vi "Stream Waveforms.vi"(9 "Stop":bool, 10 "Waveform Paths":string[](array[string])=["Targets/Controller/Hardware/Chassis/DAQ/PXI1Slot2/Analog Input/AI0", "Targets/Controller/Hardware/Chassis/DAQ/PXI1Slot2/Analog Input/AI1", "Targets/Controller/Hardware/Chassis/DAQ/PXI1Slot2/Analog Input/AI2", "Targets/Controller/Hardware/Chassis/DAQ/PXI1Slot2/Analog Input/AI3"]) -> (0 "error out":errorcluster={"status"=TRUE, "code"=-2501, "source"="TDMS Close in Stream Waveforms.vi"})   [LabVIEW 2015]
uses:
  NationalInstruments.VeriStand.ClientAPI
  <vilib>/NI Veristand/Execution/Workspace/NI VeriStand - Set Single Channel Value.vi
  <vilib>/NI Veristand/Execution/WaveformStreaming/NI_VS Waveform Streaming Interface.lvlib
  <vilib>/Analysis/NI_AALBase.lvlib
  <vilib>/NI Veristand/Execution/Workspace/NI_VS Workspace ExecutionAPI.lvlib
panel:
  in  "Waveform Task Trigger Channel":string="Targets/Controller/Hardware/Chassis/DAQ/Waveform Tasks/DAQ1/Triggers/Start Trigger"
  out "data":waveform(dbl)[](graph)
  in  "Samples to View":i64(slide)=1010 scale=300000.0..4000000.0
  in  "Offset":i64=100
  in  "Log File Path":path=path "c:/logs/log.tdms"
  out "AI2 Samples":u64
  out "AI2 offset from start (samples)":u64
  out "AI1 Samples":u64
  out "AI1 offset from start (samples)":u64
  out "AI0 Samples":u64
  out "AI0 offset from start (samples)":u64
  out "AI3 Samples":u64
  out "AI3 offset from start (samples)":u64
  out "Loop Rate Histogram":T1(graph)={"X Values"=[0.20333589539806454, 0.6100044137911523, 1.0166729321842403, 1.423341450577328, 1.830009968970416, 2.2366784873635037, 2.6433470057565915, 3.0500155241496794, 3.456684042542767, 3.863352560935855, 4.270021079328943, 4.6766895977220315, 5.08335811611512, 5.490026634508208, 5.896695152901296, 6.303363671294385, 6.710032189687473, 7.116700708080561, 7.523369226473649, 7.930037744866738, 8.336706263259826, 8.743374781652914, 9.150043300046002, 9.55671181843909, 9.963380336832179, 10.370048855225267, 10.776717373618355, 11.183385892011444, 11.590054410404532, 11.99672292879762, 12.403391447190709, 12.810059965583797, 13.216728483976885, 13.623397002369973, 14.030065520763062, 14.43673403915615, 14.843402557549238, 15.250071075942326, 15.656739594335415, 16.063408112728503, 16.47007663112159, 16.876745149514676, 17.283413667907762, 17.69008218630085, 18.096750704693935, 18.503419223087022, 18.91008774148011, 19.316756259873195, 19.72342477826628, 20.130093296659368], "Histogram: h(x)"=[1, 0, 0, 0, 0, 0, 0, 0, 0, 0, 0, 0, 0, 0, 0, 0, 0, 0, 0, 0, 0, 0, 0, 1, 0, 0, 1, 0, 0, 0, 1, 2, 3, 2, 1, 4, 4, 2, 1, 2, 0, 4, 2, 7, 7, 10, 8, 37, 248, 438]}
  out "Elapsed time":dbl
  out "Loop Rate (Hz)":dbl=19.610227107632454
  # "1. Run this VI after the VeriStand Engine is running on the target."
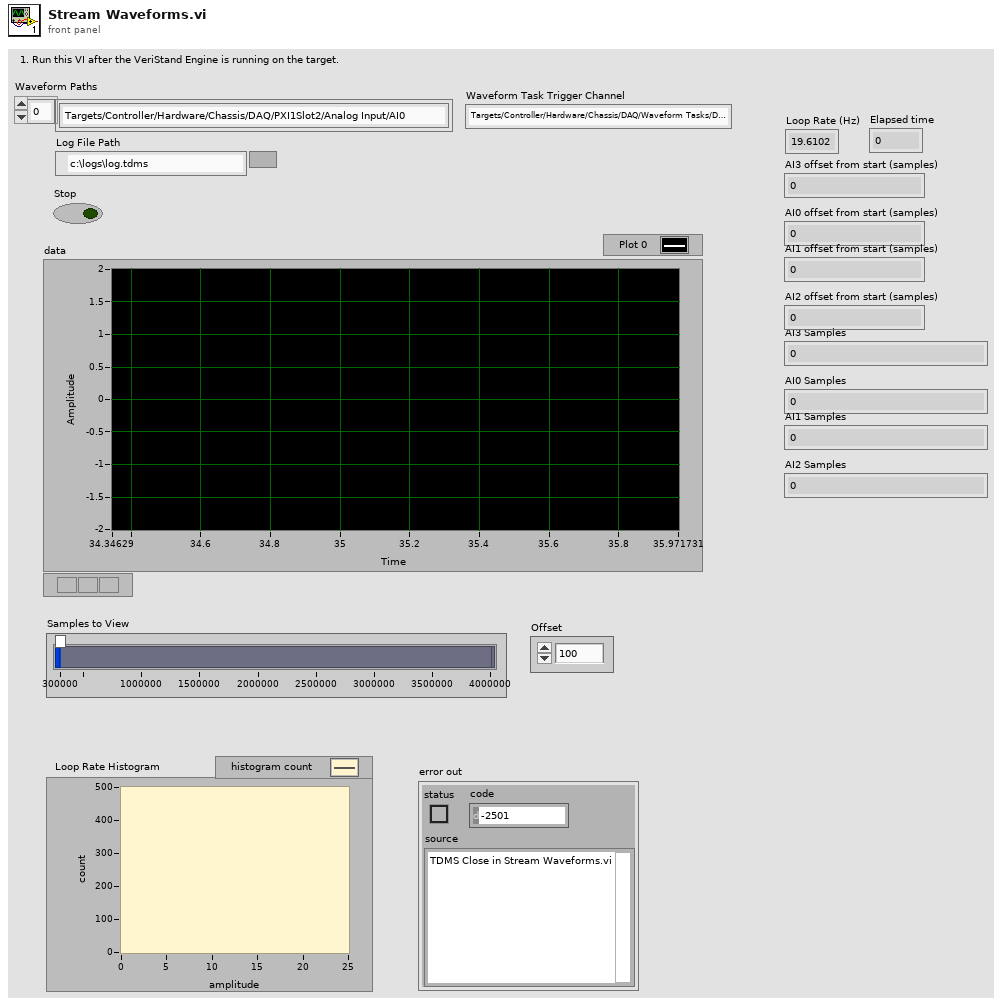
[diagram p1: front panel]
types:
  T1 = cluster{"X Values":dbl[], "Histogram: h(x)":i32[]}
  T2 = enum16{"open", "open or create", "create or replace", "create", "open (read-only)"}
  T3 = typedef "NI_VS Workspace ExecutionAPI.lvlib/WorkspaceAPI.ctl" = refnum<k24>
  T4 = typedef "NI_VS Waveform Streaming Interface.lvlib/WaveformStreamSpecification.ctl" = refnum<k24>
  T5 = typedef "NI_VS Waveform Streaming Interface.lvlib/WaveformStreamingAPI.ctl" = refnum<k24>
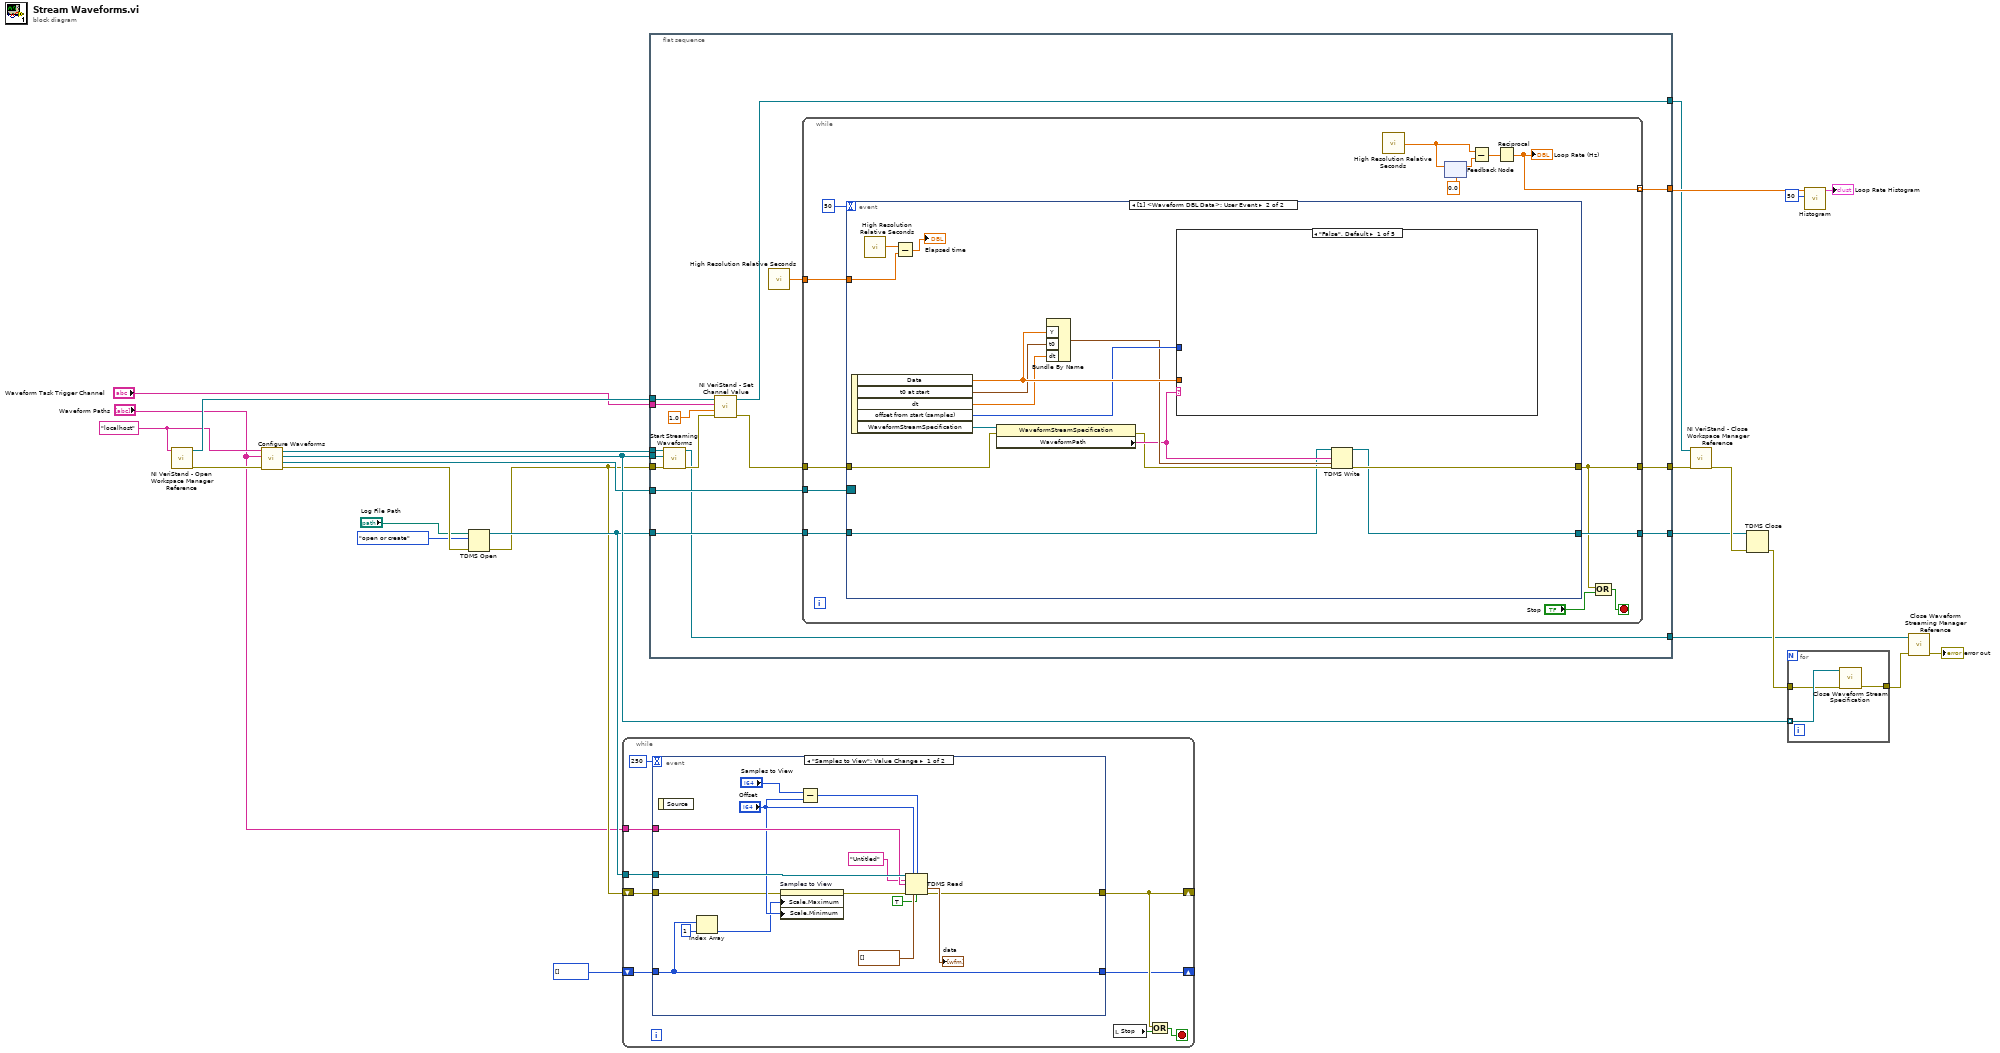
[diagram p0: block diagram]
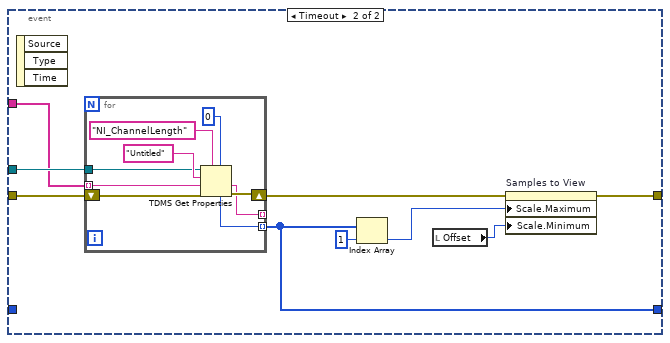
[diagram p2: hidden frame]
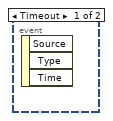
[diagram p3: hidden frame]
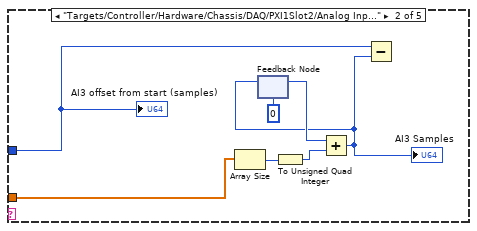
[diagram p4: hidden frame]
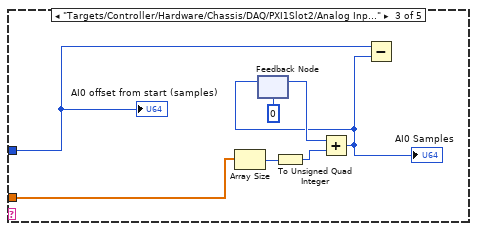
[diagram p5: hidden frame]
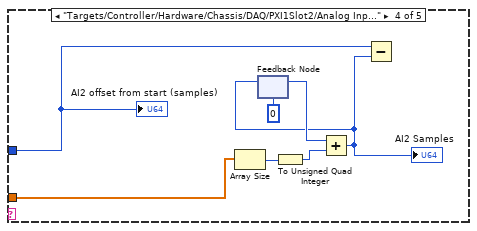
[diagram p6: hidden frame]
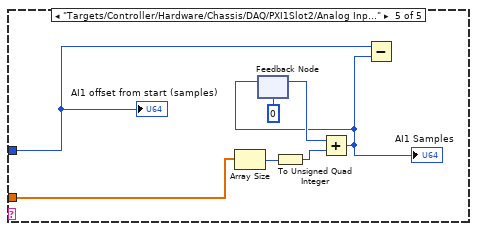
[diagram p7: hidden frame]
diagram:
  w16 = "localhost" ("Gateway IP Address (\"\": localhost)")
  n1 = call <vilib>:"NI VeriStand - Open Workspace Manager Reference.vi"("Gateway IP Address (\"\": localhost)"=w16) -> ("error out"=w17:errorcluster, "WorkspaceManager"=w20:T3)  [unwired: 9 in]
  n2 = call "Configure Waveforms.vi"("error in (no error)"=w17, "Waveform paths"="Waveform Paths", "Gateway IP Address (\"\": localhost)"=w16) -> ("error out"=w12:errorcluster, "waveform data event registration (DBL)"=w14:refnum<event-registration>, "WaveformStreamSpecifications"=w13:T4[], "WaveformStreaming out"=w15:T5)  [unwired: 5 in]
  n3 = TDMS Open(8:w12, 10:T2."open or create" ("operation (0:open)"), 11:"Log File Path") -> (0:w3:errorcluster, 3:w4:refnum<k34>)  [unwired: 4 in]
  n4 = while {
    tunnel: w4 -> [w34]
    tunnel: "Waveform Paths" -> [w33]
    shift-right: [w28] -> _
    shift-left: w3 -> [w32]
    shift-right: [w26] -> _
    shift-left: u64[] [] -> [w31]
    stop <- w30 stop-if-true
    n5 = event shown="[0] \"Samples to View\": Value Change" {
      selector: _ -> [_ _]
      dyn-events: _ -> [_ _]
      timeout: 250 -> [_ _]
      tunnel: w34 -> [w49 w57]
      tunnel: w33 -> [w48 w56]
      tunnel: w32 -> [w44 w58]
      tunnel: w31 -> [w35 _]
      tunnel: [w37 w52] -> w28
      tunnel: [w35 w54] -> w26
      event "Samples to View": Value Change {
        n6 = event-data() -> ()  [unwired: 1 in, 1 out]
        n7 = Index Array(array=w35, index=1) -> (element=w42:u64)
        n8 = property on="Samples to View" class="Slide (strict)"(error in=w44, "Scale.Maximum"=w42, "Scale.Minimum"="Offset") -> (error out=w43:errorcluster)  [unwired: 1 in, 1 out]
        n9 = Subtract(x="Samples to View", y="Offset") -> (x-y=w46:i64)
        n10 = TDMS Read(0:w49, 1:"Offset", 2:w46, 5:"Untitled" ("group name in"), 7:w48, 11:w43, 12:waveform(dbl)[] [] ("data type"), 13:TRUE ("return channels in file order? (F)")) -> (10:→"data":waveform(dbl)[], 15:w37:errorcluster)  [unwired: 4 out]
      }
      event Timeout {
        n11 = event-data() -> ()  [unwired: 1 in, 3 out]
        n12 = for {
          tunnel: [w64] -> w54 mode=indexing
          shift-right: [w65] -> w53
          shift-left: w58 -> [w63]
          tunnel: w56 -> [w62] mode=indexing
          tunnel: [w61] -> _ mode=indexing
          tunnel: w57 -> [w59]
          n13 = TDMS Get Properties(5:u64 0, 7:"NI_ChannelLength" ("property name"), 8:w63, 9:w62, 10:"Untitled" ("group name"), 11:w59) -> (0:w65:errorcluster, 1:w61:string, 4:w64:u64)  [unwired: 3 out]
        }
        n14 = Index Array(array=w54, index=1) -> (element=w51:u64)
        n15 = local read "Offset"() -> (w50:i64)
        n16 = property on="Samples to View" class="Slide (strict)"(error in=w53, "Scale.Maximum"=w51, "Scale.Minimum"=w50) -> (error out=w52:errorcluster)  [unwired: 1 in, 1 out]
      }
    }
    n17 = local read "Stop"() -> (w29:bool)
    n18 = Or(x=w28, y=w29) -> (x .or. y?=w30:bool)
  }
  n19 = flat-sequence {
    tunnel: [w82] -> w23
    tunnel: w14 -> [w83]
    tunnel: w3 -> [w80]
    tunnel: w15 -> [w79]
    tunnel: w20 -> [w77]
    tunnel: [w76] -> w19
    tunnel: "Waveform Task Trigger Channel" -> [w75]
    tunnel: w13 -> [w72]
    tunnel: w4 -> [w71]
    tunnel: [w70] -> w7
    tunnel: [w69] -> w9
    tunnel: [w68] -> w5
    frame #0 {
      n20 = call <vilib>:"Start Streaming Waveforms.vi"("error in (no error)"=w80, "WaveformStreamSpecifications"=w72, "WaveformStreaming in"=w79) -> ("error out"=w73:errorcluster, "WaveformStreaming out"=w68:T5)  [unwired: 7 in]
      n21 = call-poly <vilib>:"NI VeriStand - Set Channel Value.vi"("error in (no error)"=w73, "Value"=1.0, "Channel"=w75, "WorkspaceManager in"=w77) -> ("error out"=w78:errorcluster, "WorkspaceManager out"=w76:T3)  [unwired: 6 in]
      n22 = call <vilib>:"High Resolution Relative Seconds.vi"() -> ("relative seconds"=w81:dbl)
      n23 = while {
        tunnel: w83 -> [w97]
        tunnel: w81 -> [w92]
        tunnel: [w91] -> w82 mode=indexing
        tunnel: w78 -> [w87]
        tunnel: w71 -> [w86]
        tunnel: [w84] -> w69
        tunnel: [w85] -> w70
        stop <- w88 stop-if-true
        n24 = event shown="[1] <Waveform DBL Data>: User Event" {
          selector: w97 -> [_ _]
          dyn-events: _ -> [_ _]
          timeout: 50 -> [_ _]
          tunnel: w87 -> [_ w112]
          tunnel: w92 -> [_ w110]
          tunnel: w86 -> [_ w100]
          tunnel: [_ w99] -> w84
          tunnel: [_ w98] -> w85
          event Timeout {
            n25 = event-data() -> ()  [unwired: 1 in, 3 out]
          }
          event User Event {
            n26 = event-data() -> ("Data"=w107:dbl[], "t0 at start"=w106:timestamp, "dt"=w104:dbl, "offset from start (samples)"=w105:u64, "WaveformStreamSpecification"=w109:T4)  [unwired: 1 in]
            n27 = call <vilib>:"High Resolution Relative Seconds.vi"() -> ("relative seconds"=w111:dbl)
            n28 = Subtract(x=w111, y=w110) -> (x-y=→"Elapsed time":dbl)
            n29 = property class="WaveformStreamSpecification"(reference=w109, error in=w112) -> (error out=w101:errorcluster, "WaveformPath"=w102:string)  [unwired: 1 out]
            n30 = Bundle By Name("Y"=w107, "t0"=w106, "dt"=w104) -> (w103:waveform(dbl))  [unwired: 1 in]
            n31 = case shown="\"False\", Default" w102 {
              tunnel: w107 -> [_ w113 w120 w127 w134]
              tunnel: w105 -> [_ w115 w122 w129 w136]
              frame "False", Default {
              }
              frame "Targets/Controller/Hardware/Chassis/DAQ/PXI1Slot2/Analog Input/AI3" {
                n32 = Array Size(array=w113) -> (size(s)=w117:i32)
                n33 = feedback #1(u64 0) -> (w119:u64)
                n34 = To Unsigned Quad Integer(1:w117) -> (0:w116:u64)
                n35 = Add(x=w119, y=w116) -> (x+y=w114:u64)
                "AI3 Samples" <- w114
                n36 = feedback-in #1(w114) -> ()
                n37 = Subtract(x=w115, y=w114) -> ()  [unwired: 1 out]
                "AI3 offset from start (samples)" <- w115
              }
              frame "Targets/Controller/Hardware/Chassis/DAQ/PXI1Slot2/Analog Input/AI0" {
                n38 = Array Size(array=w120) -> (size(s)=w124:i32)
                n39 = feedback #2(u64 0) -> (w126:u64)
                n40 = To Unsigned Quad Integer(1:w124) -> (0:w123:u64)
                n41 = Add(x=w126, y=w123) -> (x+y=w121:u64)
                "AI0 Samples" <- w121
                n42 = feedback-in #2(w121) -> ()
                n43 = Subtract(x=w122, y=w121) -> ()  [unwired: 1 out]
                "AI0 offset from start (samples)" <- w122
              }
              frame "Targets/Controller/Hardware/Chassis/DAQ/PXI1Slot2/Analog Input/AI2" {
                n44 = Array Size(array=w127) -> (size(s)=w131:i32)
                n45 = feedback #3(u64 0) -> (w133:u64)
                n46 = To Unsigned Quad Integer(1:w131) -> (0:w130:u64)
                n47 = Add(x=w133, y=w130) -> (x+y=w128:u64)
                "AI2 Samples" <- w128
                n48 = feedback-in #3(w128) -> ()
                n49 = Subtract(x=w129, y=w128) -> ()  [unwired: 1 out]
                "AI2 offset from start (samples)" <- w129
              }
              frame "Targets/Controller/Hardware/Chassis/DAQ/PXI1Slot2/Analog Input/AI1" {
                n50 = Array Size(array=w134) -> (size(s)=w138:i32)
                n51 = feedback #4(u64 0) -> (w140:u64)
                n52 = To Unsigned Quad Integer(1:w138) -> (0:w137:u64)
                n53 = Add(x=w140, y=w137) -> (x+y=w135:u64)
                "AI1 Samples" <- w135
                n54 = feedback-in #4(w135) -> ()
                n55 = Subtract(x=w136, y=w135) -> ()  [unwired: 1 out]
                "AI1 offset from start (samples)" <- w136
              }
            }
            n56 = TDMS Write(0:w100, 7:w102, 9:w103, 11:w101) -> (4:w98:refnum<k34>, 15:w99:errorcluster)  [unwired: 2 in, 2 out]
          }
        }
        n57 = call <vilib>:"High Resolution Relative Seconds.vi"() -> ("relative seconds"=w93:dbl)
        n58 = feedback-in #5(w93) -> ()
        n59 = feedback #5(0.0 ("millisecond timer value")) -> (w94:dbl)
        n60 = Subtract(x=w93, y=w94) -> (x-y=w95:dbl)
        n61 = Reciprocal(x=w95) -> (1/x=w91:dbl)
        "Loop Rate (Hz)" <- w91
        n62 = Compound Arithmetic op=OR(w84, "Stop") -> (w88:bool)
      }
    }
  }
  n63 = call <vilib>:"NI VeriStand - Close Workspace Manager Reference.vi"("error in (no error)"=w9, "WorkspaceManager"=w19) -> ("error out"=w8:errorcluster)  [unwired: 9 in]
  n64 = TDMS Close(8:w8, 11:w7) -> (0:w6:errorcluster)  [unwired: 1 out]
  n65 = for {
    tunnel: [w143] -> w25
    tunnel: w13 -> [w142] mode=indexing
    tunnel: w6 -> [w141]
    n66 = call <vilib>:"Close Waveform Stream Specification.vi"("error in (no error)"=w141, "WaveformStreamSpecification"=w142) -> ("error out"=w143:errorcluster)  [unwired: 9 in]
  }
  n67 = call <vilib>:"Histogram.vi"("intervals"=50, "X"=w23) -> ("Histogram Graph"=→"Loop Rate Histogram":T1)  [unwired: 6 in, 3 out]
  n68 = call <vilib>:"Close Waveform Streaming Manager Reference.vi"("error in (no error)"=w25, "WaveformStreaming"=w5) -> ("error out"=→"error out":errorcluster)  [unwired: 9 in]
